vi "Copy i_th image to array v2.vi"(0 "Img Array In":T1[](array[typedef]), 7 "Image Src":T1, 11 "error in (no error)":errorcluster, 13 "Index":i32) -> (4 "Img Array Out":T1[](array[typedef]), 15 "error out":errorcluster)   [LabVIEW 2013]
uses:
  <vilib>/vision/Image Controls.llb/IMAQ Image.ctl
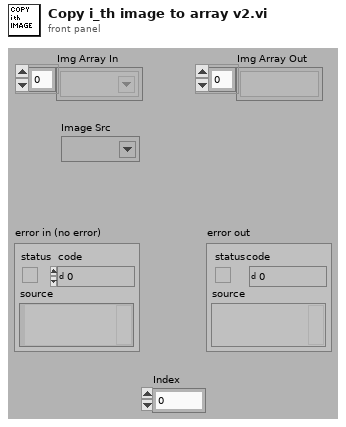
[diagram p1: front panel]
types:
  T1 = typedef "IMAQ Image.ctl" = refnum<image>
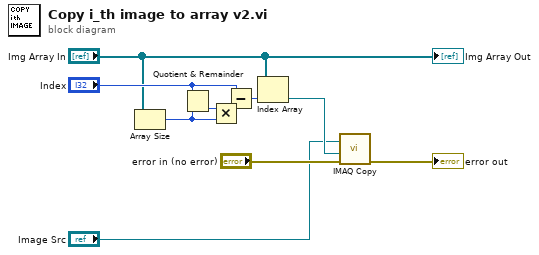
[diagram p0: block diagram]
diagram:
  n1 = Array Size(array="Img Array In") -> (size(s)=w6:i32)
  n2 = Quotient & Remainder(x="Index", y=w6) -> (floor(x/y)=w7:i32)  [unwired: 1 out]
  n3 = Multiply(x=w7, y=w6) -> (x*y=w9:i32)
  n4 = Subtract(x="Index", y=w9) -> (x-y=w10:i32)
  n5 = Index Array(array="Img Array In", index=w10) -> (element=w2:T1)
  n6 = call "IMAQ Copy"("error in (no error)"="error in (no error)", "Image Dst"=w2, "Image Src"="Image Src") -> ("error out"=→"error out":errorcluster)  [unwired: 3 in, 1 out]
  "Img Array Out" <- "Img Array In"
